vi "bitfile name to item property strings.vi"(11 "Name in bitfile":string) -> (2 "Notes String":string, 3 "Reservation String":string)   [LabVIEW 2016, in "FPGA Resource Manager System Defintion.lvlib"]
uses:
  FPGA Resource Manager System Defintion.lvlib
  global constants.vi
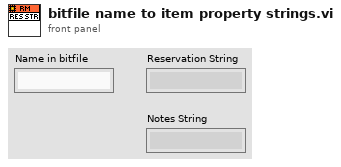
[diagram p1: front panel]
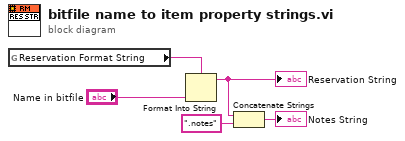
[diagram p0: block diagram]
diagram:
  n1 = global read "global constants.vi" "Reservation Format String"() -> (w5:string)
  n2 = Format Into String(format string=w5, "Name in bitfile") -> (resulting string=w3:string)  [unwired: 2 in, 1 out]
  "Reservation String" <- w3
  n3 = Concatenate Strings(w3, ".notes" ("string")) -> (→"Notes String":string)
